vi "3D_express_skeletonvi.vi"(9 "Padrão":dbl[][](array[numeric]), 10 "Body":dbl[][](array[numeric]), 11 "Scene In":refnum<vi>) -> (3 "3D Picture":refnum<vi>(3d-picture))   [LabVIEW 2016]
uses:
  <vilib>/3D Express/3D Express.lvlib
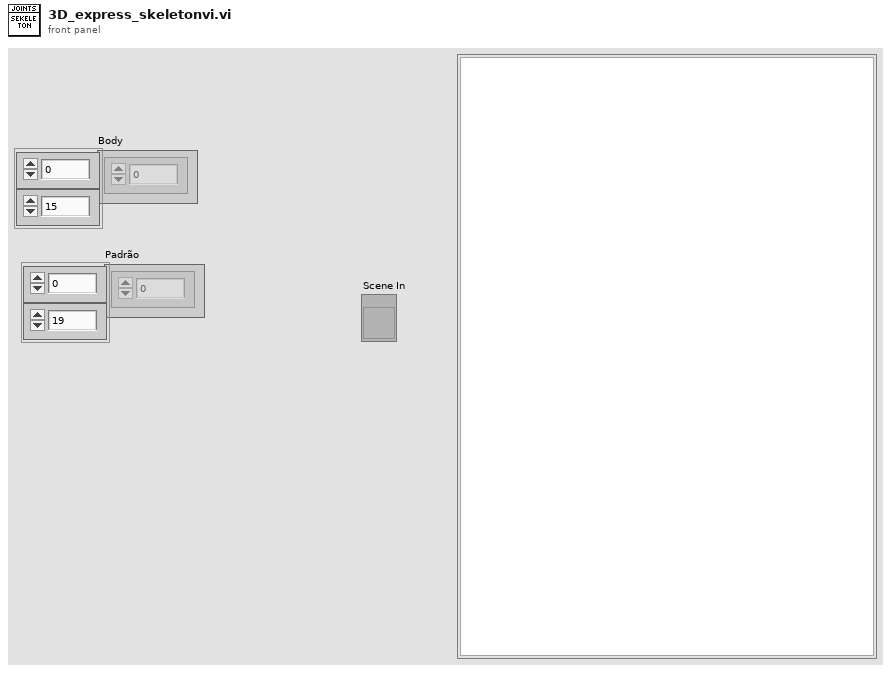
[diagram p1: front panel]
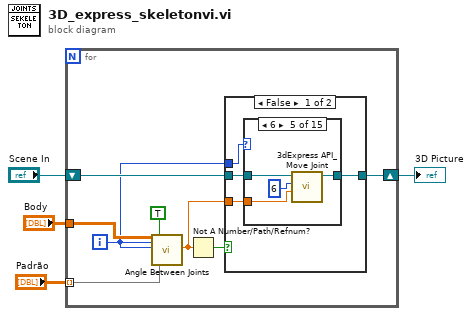
[diagram p0: block diagram]
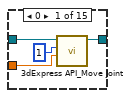
[diagram p2: hidden frame]
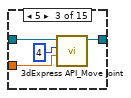
[diagram p4: hidden frame]
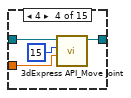
[diagram p5: hidden frame]
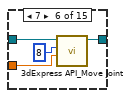
[diagram p6: hidden frame]
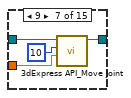
[diagram p7: hidden frame]
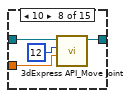
[diagram p8: hidden frame]
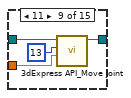
[diagram p9: hidden frame]
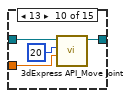
[diagram p10: hidden frame]
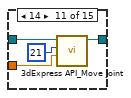
[diagram p11: hidden frame]
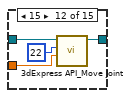
[diagram p12: hidden frame]
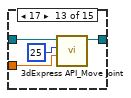
[diagram p13: hidden frame]
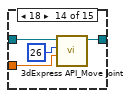
[diagram p14: hidden frame]
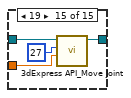
[diagram p15: hidden frame]
diagram:
  n1 = for {
    shift-right: [w8] -> w1
    shift-left: "Scene In" -> [w12]
    tunnel: "Body" -> [w9]
    tunnel: "Padrão" -> [w11] mode=indexing
    i -> [w5]
    n2 = call <vilib>:"Angle Between Joints.vi"("Array of Joint Positions"=w9, "Joint 1"=w5, "Joint 2"=w5, "Compare Vector 1-2 with User defined Vector"=TRUE, "Custom Vector"=w11) -> ("Angle Between Joints (degrees)"=w6:dbl)  [unwired: 9 in, 5 out]
    n3 = Not A Number/Path/Refnum?(number/path/refnum=w6) -> (NaN/Path/Refnum?=w7:bool)
    n4 = case shown="False" w7 {
      tunnel: w12 -> [w16 w74]
      tunnel: w6 -> [w15 _]
      tunnel: [w14 w74] -> w8
      tunnel: w5 -> [w13 _]
      frame False {
        n5 = case shown="6" w13 {
          tunnel: w16 -> [w20 w21 w25 w29 w33 w37 w41 w45 w49 w53 w57 w61 w65 w69 w73]
          tunnel: w15 -> [w19 _ w24 w28 w32 w36 w40 w44 w48 w52 w56 w60 w64 w68 w72]
          tunnel: [w18 w21 w23 w27 w31 w35 w39 w43 w47 w51 w55 w59 w63 w67 w71] -> w14
          frame 0 {
            n6 = call <vilib>:"3dExpress API_Move Joint.vi"("Joint Data"=w19, "Joint Index"=1, "Scene in"=w20) -> ("Scene out"=w18:refnum<vi>)  [unwired: 7 in, 1 out]
          }
          frame 100, Default {
          }
          frame 5 {
            n7 = call <vilib>:"3dExpress API_Move Joint.vi"("Joint Data"=w24, "Joint Index"=4, "Scene in"=w25) -> ("Scene out"=w23:refnum<vi>)  [unwired: 7 in, 1 out]
          }
          frame 4 {
            n8 = call <vilib>:"3dExpress API_Move Joint.vi"("Joint Data"=w28, "Joint Index"=15, "Scene in"=w29) -> ("Scene out"=w27:refnum<vi>)  [unwired: 7 in, 1 out]
          }
          frame 6 {
            n9 = call <vilib>:"3dExpress API_Move Joint.vi"("Joint Data"=w32, "Joint Index"=6, "Scene in"=w33) -> ("Scene out"=w31:refnum<vi>)  [unwired: 7 in, 1 out]
          }
          frame 7 {
            n10 = call <vilib>:"3dExpress API_Move Joint.vi"("Joint Data"=w36, "Joint Index"=8, "Scene in"=w37) -> ("Scene out"=w35:refnum<vi>)  [unwired: 7 in, 1 out]
          }
          frame 9 {
            n11 = call <vilib>:"3dExpress API_Move Joint.vi"("Joint Data"=w40, "Joint Index"=10, "Scene in"=w41) -> ("Scene out"=w39:refnum<vi>)  [unwired: 7 in, 1 out]
          }
          frame 10 {
            n12 = call <vilib>:"3dExpress API_Move Joint.vi"("Joint Data"=w44, "Joint Index"=12, "Scene in"=w45) -> ("Scene out"=w43:refnum<vi>)  [unwired: 7 in, 1 out]
          }
          frame 11 {
            n13 = call <vilib>:"3dExpress API_Move Joint.vi"("Joint Data"=w48, "Joint Index"=13, "Scene in"=w49) -> ("Scene out"=w47:refnum<vi>)  [unwired: 7 in, 1 out]
          }
          frame 13 {
            n14 = call <vilib>:"3dExpress API_Move Joint.vi"("Joint Data"=w52, "Joint Index"=20, "Scene in"=w53) -> ("Scene out"=w51:refnum<vi>)  [unwired: 7 in, 1 out]
          }
          frame 14 {
            n15 = call <vilib>:"3dExpress API_Move Joint.vi"("Joint Data"=w56, "Joint Index"=21, "Scene in"=w57) -> ("Scene out"=w55:refnum<vi>)  [unwired: 7 in, 1 out]
          }
          frame 15 {
            n16 = call <vilib>:"3dExpress API_Move Joint.vi"("Joint Data"=w60, "Joint Index"=22, "Scene in"=w61) -> ("Scene out"=w59:refnum<vi>)  [unwired: 7 in, 1 out]
          }
          frame 17 {
            n17 = call <vilib>:"3dExpress API_Move Joint.vi"("Joint Data"=w64, "Joint Index"=25, "Scene in"=w65) -> ("Scene out"=w63:refnum<vi>)  [unwired: 7 in, 1 out]
          }
          frame 18 {
            n18 = call <vilib>:"3dExpress API_Move Joint.vi"("Joint Data"=w68, "Joint Index"=26, "Scene in"=w69) -> ("Scene out"=w67:refnum<vi>)  [unwired: 7 in, 1 out]
          }
          frame 19 {
            n19 = call <vilib>:"3dExpress API_Move Joint.vi"("Joint Data"=w72, "Joint Index"=27, "Scene in"=w73) -> ("Scene out"=w71:refnum<vi>)  [unwired: 7 in, 1 out]
          }
        }
      }
      frame True {
      }
    }
  }
  "3D Picture" <- w1
